vi "SimpleRamp_Generate_v4.vi"(4 "error in (no error)":errorcluster, 5 "Error Locator":string, 6 "formula":string="sin(10*f)", 7 "Current Variable settings":T1[](array[typedef]), 8 "dt":dbl=1.0, 9 "Points":u32=500) -> (0 "error out":errorcluster, 1 "x values":dbl[](array[numeric]), 2 "y values":dbl[](array[numeric]))   [LabVIEW 2013]
doc: "Evaluate expressions on Ramp line which include timing infomation (f,t,dt,tMax). Current Variable settings are optional as they are known by the Lua state if already set prior."
uses:
  TypeDefs/Active procedure variables.ctl
  PackedLibraries/LuaEvaluatorAPI.lvlibp/API/t_Caching_Expression_Evaluator_Methods_Table.ctl
  PackedLibraries/LuaEvaluatorAPI.lvlibp
  Globals/UserFunctions.vi
panel:
  # "This computes the expression, where\n\"f\" on the domain [0,1]\nor\n\"t\" varaible is in absolute units."
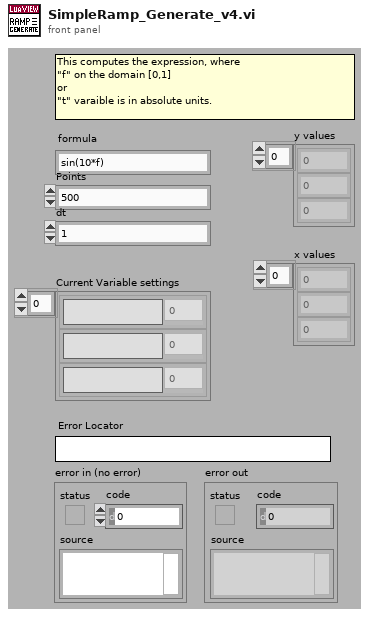
[diagram p1: front panel]
types:
  T1 = typedef "Active procedure variables.ctl" = cluster{"Procedure variable":string, "Value":dbl}
  T2 = typedef "LuaEvaluatorAPI.lvlibp/t_Caching_Expression_Evaluator_Methods_Table.ctl" = enum16{"set", "get", "eval", "assign", "isvalid", "execute", "evaltable", "close"}
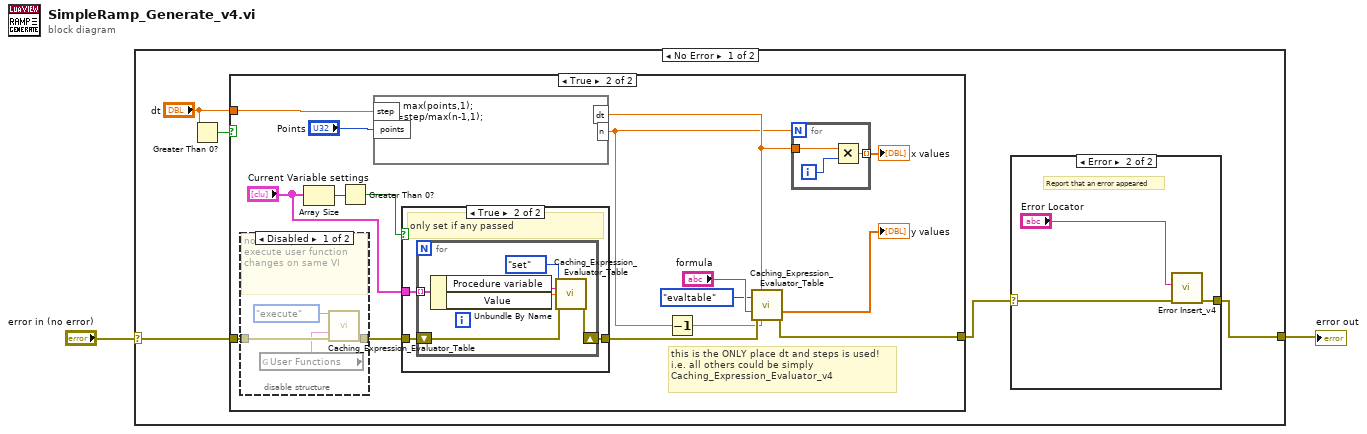
[diagram p0: block diagram]
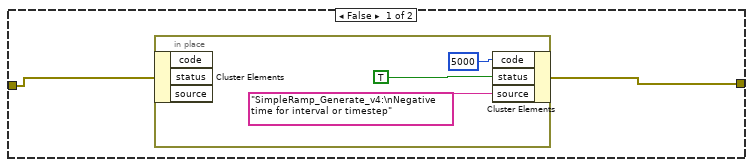
[diagram p3: hidden frame]
diagram:
  n1 = case shown="No Error" "error in (no error)" {
    selector: "error in (no error)" -> [w7 w50]
    tunnel: [w3 w50] -> w1
    frame No Error {
      n2 = Greater Than 0?(x="dt") -> (x > 0?=w5:bool)
      n3 = case shown="True" w5 {
        tunnel: [w12 w31] -> w4
        tunnel: w7 -> [w13 w26]
        tunnel: "dt" -> [_ w23]
        frame False {
          n4 = in-place {
            n5 = in-place-cluster #1(w13) -> ()  [unwired: 3 out]
            n6 = in-place-cluster #1("code"=5000, "status"=TRUE, "source"="SimpleRamp_Generate_v4:\nNegative time for interval or timestep") -> (w12:errorcluster)
          }
        }
        frame True {
          # "this is the ONLY place dt and steps is used!\ni.e. all others could be simply\nCaching_Expression_Evaluator_v4"
          n7 = disable-structure shown="Disabled" {
            disable-tunnel: [w46 _] -> w27
            disable-tunnel: w26 -> [w45 _]
            frame Disabled {
              # "no need! provided we execute user function changes on same VI"
              n8 = global read "UserFunctions.vi" "User Functions"() -> (w44:string)
              n9 = call "Caching_Expression_Evaluator_Table.vi"("method"=t_Caching_Expression_Evaluator_Methods_Table."execute", "expression/scriptlet"=w44, "error in (no error)"=w45) -> ("error out"=w46:errorcluster)  [unwired: 4 in, 8 out]
            }
            frame Enabled {
            }
          }
          n10 = Array Size(array="Current Variable settings") -> (size(s)=w18:i32)
          n11 = Greater Than 0?(x=w18) -> (x > 0?=w17:bool)
          n12 = formula code="n = max(points,1);\ndt =step/max(n-1,1);"("points"="Points", "step"=w23) -> ("dt"=w25:dbl, "n"=w22:dbl)
          n13 = case shown="True" w17 {
            tunnel: [w33 w36] -> w32
            tunnel: "Current Variable settings" -> [_ w35]
            tunnel: w27 -> [w33 w34]
            frame False {
            }
            frame True {
              # "only set if any passed"
              n14 = for {
                shift-right: [w42] -> w36
                shift-left: w34 -> [w41]
                tunnel: w35 -> [w38] mode=indexing
                n15 = Unbundle By Name(w38) -> ("Procedure variable"=w40:string, "Value"=w39:dbl)
                n16 = call "Caching_Expression_Evaluator_Table.vi"("method"=t_Caching_Expression_Evaluator_Methods_Table."set", "variable"=w40, "value in"=w39, "error in (no error)"=w41) -> ("error out"=w42:errorcluster)  [unwired: 3 in, 8 out]
              }
            }
          }
          n17 = Decrement(x=w22) -> (x-1=w21:dbl)
          n18 = call "Caching_Expression_Evaluator_Table.vi"("method"=t_Caching_Expression_Evaluator_Methods_Table."evaltable", "dt (for table)"=w25, "expression/scriptlet"="formula", "error in (no error)"=w32, "steps (for table)"=w21) -> ("table out"=→"y values":dbl[], "error out"=w31:errorcluster)  [unwired: 2 in, 7 out]
          n19 = for {
            N: w22 -> [_]
            tunnel: w25 -> [w49]
            tunnel: [w47] -> w28 mode=indexing
            i -> [w48]
            n20 = Multiply(x=w49, y=w48) -> (x*y=w47:dbl)
          }
          "x values" <- w28
        }
      }
      n21 = case shown="Error" w4 {
        selector: w4 -> [w8 w11]
        tunnel: [w8 w10] -> w3
        frame No Error {
        }
        frame Error {
          # "Report that an error appeared"
          n22 = call "Error Insert_v4.vi"("error in (no error)"=w11, "error message (\"\")"="Error Locator") -> ("error out"=w10:errorcluster)  [unwired: 1 in, 6 out]
        }
      }
    }
    frame Error {
    }
  }
  "error out" <- w1
